vi "Pendulum Sequence.vi"() -> ()   [LabVIEW 2018]
uses:
  Model/Target.ctl
  <vilib>/Simulation/Scripting/Companion Diagram/SimConfigNode/SimParams.ctl
  <vilib>/Simulation/Scripting/Companion Diagram/SimConfigNode/_simSolvers.ctl
  <vilib>/Simulation/Implementation/Shared/SIMSCR Execution Mode.ctl
  <vilib>/Simulation/Param Hierarchy/Typedefs/SIMPH Param Control Actions.ctl
  <vilib>/Simulation/Implementation/Shared/NILVSim_ParamChanged.vi
  <vilib>/Simulation/Implementation/Shared/NILVSIM_BeginStep.vi
  <vilib>/Simulation/Implementation/Shared/NILVSim_Manager.vi
  <vilib>/Utility/error.llb/Clear Errors.vi
  <vilib>/Simulation/Implementation/Shared/NILVSim_FinalizeModel.vi
  <vilib>/Simulation/Implementation/Shared/SIM Unbundle Sim Info.vi
  <vilib>/Simulation/Implementation/Shared/NILVSim_Initialize.vi
  <vilib>/Simulation/Utility/Implementation/NILVSim Get Time and IsAcceptedStep.vi
  <vilib>/Simulation/Implementation/Shared/SIMSH Read Queue.vi
  <vilib>/Simulation/Implementation/Shared/NILVSim_GetModelError.vi
  <vilib>/Simulation/Implementation/Shared/SIM Bundle Sim Info.vi
  <vilib>/Simulation/Scripting/Companion Diagram/SimConfigNode/SimDog.xnode
  Model/Cart Pendulum Model.vi
  <vilib>/Simulation/Implementation/XNodeFramework/SimXNode/SimX.xnode
  <vilib>/Simulation/Implementation/Shared/NI_SIM_Implementation.lvlib
panel:
  out "States":dbl[](array[numeric]) format="%.4f"
  out "In Range?":bool
  out "In Range Seconds":dbl format="%.2f"
  out "Done":bool
  out "Off Track":bool
  out "Pendulum":picture
  out "Target":T1 {"Position" min=-0.5 max=0.5 step=0.1 format="%.2g"}
  out "Seconds":dbl format="%.3f"
  in  "stop":bool
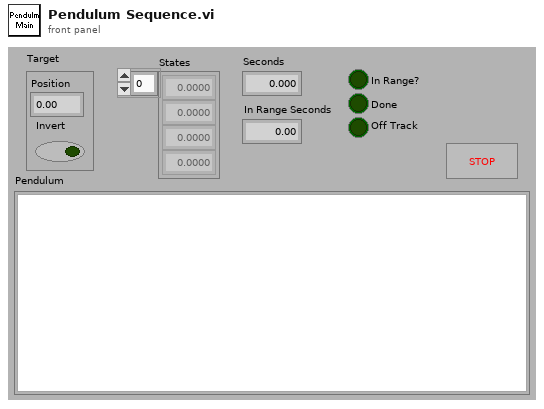
[diagram p1: front panel]
types:
  T1 = typedef "Target.ctl" = cluster{"Position":dbl, "Invert":bool}
  T2 = enum16{"Random", "List 1", "List 2", "List 3", "List 4", "List 5"}
  T3 = typedef "SIMSCR Execution Mode.ctl" = enum16{"Simulate to Completion", "Single Time-Step Simulation (Fixed Step Only)"}
  T4 = typedef "SIMPH Param Control Actions.ctl" = enum16{"get params", "set params"}
  T5 = cluster{"SIMSH Sim Time":dbl, "Integrator 3":cluster{"output":dbl[]}, "Build Array":cluster{"appended array":dbl[]}, "Index Array":cluster{"element":dbl}, "Negate 2":cluster{"-x":dbl}, "Negate":cluster{"-x":dbl}, "Sine & Cosine":cluster{"sin(x)":dbl, "cos(x)":dbl}, "Formula Node":cluster{"dx":dbl, "ddx":dbl, "dT":dbl, "ddT":dbl}}
  T6 = typedef "SimParams.ctl" = cluster{"Initial Time (s)":dbl, "Final Time (s)":dbl, "Step Size (s)":dbl, "ODE Solver":T7, "Minimum Step Size (s)":dbl, "Maximum Step Size (s)":dbl, "Relative Tolerance":dbl, "Absolute Tolerance":dbl, "Software Timing":bool, "Initial Step Size (s)":dbl, "Automatic Fixed Step Size?":bool, "Automatic Discrete Step Size?":bool, "Discrete Step Size (s)":dbl, "Calculate using Time Step":bool, "Solver Wired?":bool, "Prev.Frm.Expected End":u64, "Prev.Frm.Actual End":u64, "Prev.Frm.Finished Late?":bool, "Prev.Iter.Expected End":u64, "Prev.Iter.Actual End":u64, "Prev.Iter.Finished Late?":bool, "Expected Iteration Start":u64, "Actual Iteration Start":u64, "Expected Frame Start":u64, "Actual Frame Start":u64, "Source Name":string, "Name":string, "Period":i64, "Deadline":i64, "Offset":i64, "Start":i64, "Priority":i32, "Timeout":i32, "Processor":i32, "Mode":enum32{"No Change", "Process missed periods, maintain original phase", "Discard missed periods, maintain original phase", "Process missed periods, ignore original phase", "Discard missed periods, ignore original phase"}, "Wakeup reason":enum32{"Normal", "Aborted", "Asynchronous wakeup", "Timing source error", "Timed loop error", "Timeout"}, "Error":errorcluster, "Source Type":string, "Secondary Source Type":string, "Global End Time":u64, "Global Start Time":u64, "Full Solver Reset":bool, "Execution Mode":T3, "Nan/Inf Check":bool, "Custom Solver Library":string, "Solver Is Variable":bool, "custom solver name":string, "Signal Collection Decimation":u32}
  T7 = typedef "_simSolvers.ctl" = enum16{"Runge-Kutta 1 (Euler)", "Runge-Kutta 2", "Runge-Kutta 3", "Runge-Kutta 4", "Runge-Kutta 23 (variable)", "Runge-Kutta 45 (variable)", "BDF (variable)", "Adams-Moulton (variable)", "Rosenbrock (variable)", "Discrete States Only", "SDIRK 4 (variable)", "Radau 5 (variable)", "Radau 9 (variable)", "Radau 13 (variable)", "Radau [Variable Order] (variable)", "Gear's Method (variable)", "Linearizer", "State Query", "Trim Eval", "Custom Solver"}
  T8 = typedef "States.ctl" = dbl[]
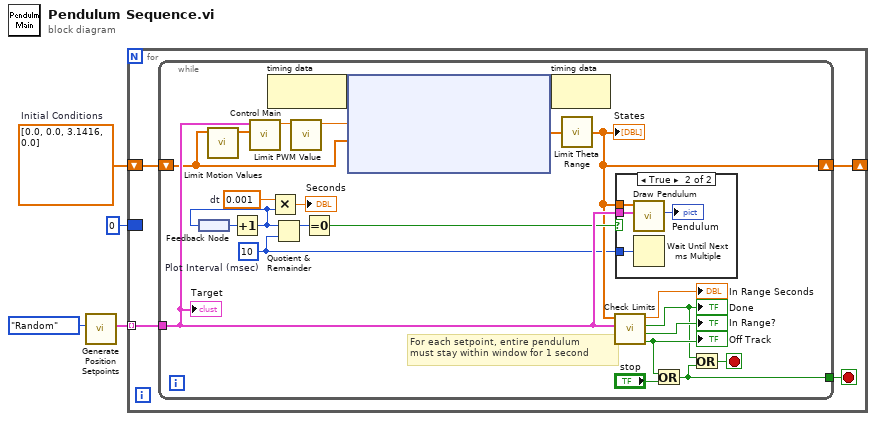
[diagram p0: block diagram]
diagram:
  w4 = dbl[] [0.0, 0.0, 3.1416, 0.0]  # Initial Conditions
  n1 = call "Generate Position Setpoints.vi"("Select List"=T2."Random") -> ("Targets"=w2:T1[])  [unwired: 10 in]
  n2 = for {
    tunnel: w2 -> [w8] mode=indexing
    shift-right: [w5] -> _
    shift-left: w4 -> [w6]
    border: u32 0 -> [_]
    stop <- w7 stop-if-true
    n3 = while {
      tunnel: w8 -> [w20]
      tunnel: [w26] -> w7
      shift-right: [w15] -> w5
      shift-left: w6 -> [w10]
      stop <- w28 stop-if-true
      w14 = u32 10  # Plot Interval (msec)
      w25 = 0.001  # dt
      # "For each setpoint, entire pendulum\nmust stay within window for 1 second"
      n4 = feedback #1() -> (w29:u32)
      n5 = call "Limit Motion Values.vi"("States In"=w10) -> ("States Out"=w11:T8)  [unwired: 10 in]
      n6 = Increment(x=w29) -> (x+1=w16:u32)
      n7 = feedback-in #1(w16) -> ()
      n8 = call "Control Main.vi"("States"=w11, "Target"=w20) -> ("PWM"=w18:dbl)  [unwired: 9 in]
      n9 = node-c288() -> (w24:variant)  [unwired: 1 in]
      n10 = Multiply(x=w25, y=w16) -> (x*y=→"Seconds":dbl)
      n11 = Quotient & Remainder(x=w16, y=w14) -> (x-y*floor(x/y)=w31:u32)  [unwired: 1 out]
      n12 = call "Limit PWM Value.vi"("PWM In"=w18) -> ("PWM Out"=w17:dbl)  [unwired: 10 in]
      n13 = Equal To 0?(x=w31) -> (x = 0?=w19:bool)
      n14 = node-c254 ("Control & Simulation Loop 2")(w24, w17, w10) -> (w23:variant, w9:dbl[])
      n15 = node-c288(w23) -> ()  [unwired: 1 out]
      n16 = call "Limit Theta Range.vi"("States In"=w9) -> ("States Out"=w15:T8)
      "States" <- w15
      n17 = call "Check Limits.vi"("Target"=w20, "States"=w15) -> ("Off Track"=w13:bool, "In Range"=→"In Range?":bool, "Done"=w12:bool, "In Range Seconds"=→"In Range Seconds":dbl)  [unwired: 2 in, 1 out]
      "Done" <- w12
      "Off Track" <- w13
      n18 = case shown="True" w19 {
        tunnel: w20 -> [_ w268]
        tunnel: w15 -> [_ w267]
        tunnel: w14 -> [_ w265]
        frame False {
        }
        frame True {
          n19 = call "Draw Pendulum.vi"("Target"=w268, "States In"=w267) -> ("Picture"=→"Pendulum":picture)  [unwired: 9 in]
          n20 = Wait Until Next ms Multiple(millisecond multiple=w265) -> ()  [unwired: 1 out]
        }
      }
      n21 = Or(x=w13, y="stop") -> (x .or. y?=w26:bool)
      n22 = Or(x=w12, y=w26) -> (x .or. y?=w28:bool)
      "Target" <- w20
    }
  }
